vi "Match.vi"(10 "log record":T1 {"timestamp" format="%<%x %.3X>T"}, 11 "scope in":refnum<class "Scope.lvclass">) -> (2 "matches":bool[](array[boolean]), 3 "scope out":refnum<class "Scope.lvclass">)   [LabVIEW 2024, in "Logging.lvlib" / "Scope.lvclass"]
uses:
  Scope.lvclass
  Log Record.ctl
  Logger/Internal Log Levels.ctl
  Logging.lvlib
panel:
  # "Connector Pane"
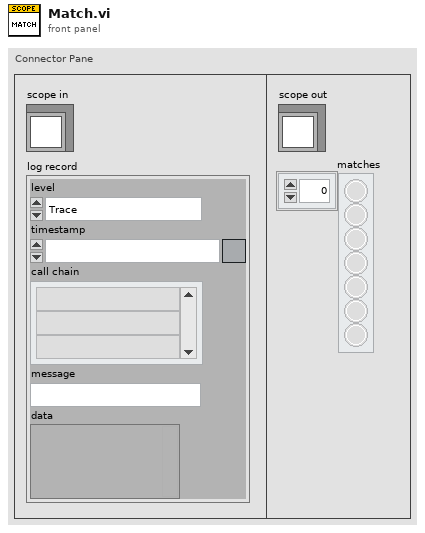
[diagram p1: front panel]
types:
  T1 = typedef "Logging.lvlib/Log Record.ctl" = cluster{"level":T2, "timestamp":timestamp, "call chain":string[], "message":string, "data":variant}
  T2 = typedef "Logging.lvlib/Internal Log Levels.ctl" = enum16{"Trace", "Debug", "Info", "Warning", "Error", "Critical", "Internal"}
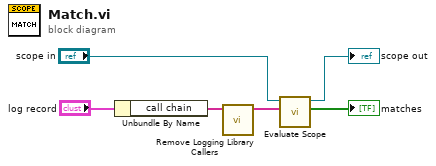
[diagram p0: block diagram]
diagram:
  n1 = Unbundle By Name("log record") -> ("call chain"=w2:string[])
  n2 = call "Remove Logging Library Callers.vi"("call chain"=w2) -> ("trimmed call chain"=w1:string[])  [unwired: 10 in]
  n3 = call-dynamic "Evaluate Scope.vi"("call chain"=w1, "scope in"="scope in") -> ("matches"=→"matches":bool[], "scope out"=→"scope out":refnum<class "Scope.lvclass">)  [unwired: 8 in]
